vi "NI-USB6343.vi"() -> ()   [LabVIEW 2020]
doc: "test"
uses:
  LabVIEW 2020 Toolkits/toolkits_lv2020_32bit/Synchronization.llb/SynchRefs_SetGet.ctl
  LabVIEW 2020 Toolkits/VI Server Toolkit/VI Server Libraries/VI Server_SetControl.llb/VI Server_BOOL_Set.vi
  LabVIEW 2020 Toolkits/VI Server Toolkit/VI Server Libraries/VI Server_Set Controls.llb/Set STR Control.vi
  LabVIEW 2020 Toolkits/VI Server Toolkit/VI Server Libraries/VI Server_GetControl.llb/VI Server_STR_Get.vi
  LabVIEW 2020 Toolkits/VI Server Toolkit/VI Server Libraries/VI Server_GetControl.llb/VI Server_DAQmx_Device_Get.vi
  LabVIEW 2020 Toolkits/VI Server Toolkit/VI Server Toolkit LV2013.lvlib
panel:
  in  "LastAction.AddToSecuence":bool
  out "System.Message":string caption="System Message"
  in  "Help":bool
  in  "FP.Hide":bool caption="FrontPanel.Hide"
  in  "EXIT":bool
  in  "Tab.Main":T1(tab)
  in  "AI.SaveGraphToFile":bool
  in  "AI.Graph.Plots":u16(ring) items=["NI-USB6343/ai0", "NI-USB6343/ai1", "NI-USB6343/ai2"]
  out "AI.WaveformGraph":waveform(dbl)[](graph) caption="Waveform Graph"
  in  "AI.MultiChannelAcquisition":bool
  in  "AI.PhysicalChannel.Include":bool
  out "AI.ActualSampleRate":dbl=1000.0 caption="Actual Sample Rate" format="%0.2f"
  out "AI.Averaged.Mesurement":dbl caption="Averaged Mesurement" format="%0.4f V"
  in  "AI.Measure":bool caption="AI:Measure"
  in  "AI.Number.Of.Samples":i32=100 caption="Number Of Samples"
  in  "AI.SampleRate":dbl=1000.0 caption="Sample Rate" format="%0.0f Hz"
  in  "AI.MinInputLimit":dbl caption="Min Input Limit" min=-10.0 max=10.0 format="%0.3f V"
  in  "AI.MaxInputLimit":dbl caption="Max Input Limit" min=-10.0 max=10.0 format="%0.3f V"
  in  "AI.TerminalConfiguration":u16(ring)=65535 caption="Terminal Configuration" items=["default"=65535, "RSE"=10083, "NRSE"=10078, "Differential"=10106, "Pseudodifferential"=12529]
  in  "AI.Sample.Mode":u16(ring)=12522 caption="Sample Mode" items=["Finite Samples"=10178, "Continuous Samples"=10123]
  in  "AI.Physical.Channel":tag="Dev1/ai0" caption="Physical Channel"
  out "AO.Update.Time":u32 caption="AO Update Time" format="%.0f msec"
  in  "AO.GenerationMode":u16(ring) caption="Generation Mode" items=["Voltage DC", "Voltage Sine Wave Generation", "Voltage Triangle Wave Generation", "Voltage Square Wave Generation", "Voltage Sawtooth Wave Generation"]
  in  "AO.Physical.Channel":tag="Dev1/ai0" caption="Physical Channel"
  in  "AO.Update":bool
  in  "AO.Output":bool caption="AO:Output"
  in  "AO.SampleMode":u16(ring) caption="Sample Mode" items=["Finite Samples"=10178, "Continious Samples"=10123]
  in  "AO.NumberOfSamples":i32=1000 caption="Number Of Samples" min=2
  in  "AO.SampleRate":dbl=1000.0 caption="Sample Rate" format="%0.1f Hz"
  in  "AO.Sample.Clock.Source":tag="OnboardClock" caption="Sample Clock Source"
  out "AO.ActualSampleRate":dbl=1000.0 caption="Actual Sample Rate" format="%0.2f"
  in  "AO.MaxVoltage":dbl=5.0 caption="Max Voltage" format="%0.3f V"
  in  "AO.MinVoltage":dbl=-5.0 caption="Min Voltage" format="%0.3f V"
  out "AO.WaveformGraph":waveform(dbl)(graph) caption="Waveform Graph"
  in  "AO.OutputVoltage":dbl(slide) caption="Amplitude" min=-10.0 max=10.0 scale=-10.0..10.0 scale format="%0.3f V"
  in  "AO.SinewaveFrequency":dbl=10.0 caption="Sinewave Frequency" format="%0.2p Hz"
  in  "DO.Port.Mask.Apply":bool caption="DO:Port.Mask.Apply"
  in  "DO.Port.Lines.31:24.Mask":u8 caption="Port&Lines 31:24" format="%08b"
  in  "DO.Port.Lines.23:16.Mask":u8 caption="Port&Lines 23:16" format="%08b"
  in  "DO.Port.Lines.15:8.Mask":u8 caption="Port&Lines 15:8" format="%08b"
  in  "DO.Port.Lines.7:0.Mask":u8 caption="Port&Lines 7:0" format="%08b"
  out "DO.Port.State.Verify":bool caption="Verified"
  out "DO.Line.State.Verify":bool caption="Verified"
  in  "DO.Line.State":bool caption="State"
  in  "DO.Line":tag="Dev1/port0/line0:7" caption="Line"
  in  "DO.Line.Update":bool caption="Update:"
  in  "DO.Port.Update":bool caption="DO:Port.Update"
  in  "DO.Port.Lines.31:24":u8 caption="Port&Lines 31:24" format="%08b"
  in  "DO.Port.Lines.23:16":u8 caption="Port&Lines 23:16" format="%08b"
  in  "DO.Port.Lines.15:8":u8 caption="Port&Lines 15:8" format="%08b"
  in  "DO.Port.Lines.7:0":u8 caption="Port&Lines 7:0" format="%08b"
  in  "DO.Port":tag="Dev1/port0/line0:7" caption="Port"
  out "DI.Line.State":bool caption="State"
  in  "DI.Port.Update":bool caption="DI:Port.Update"
  out "DI.Port.Lines.24:31":u8 caption="Port&Lines 31:24" format="%08b"
  out "DI.Port.Lines.16:23":u8 caption="Port&Lines 23:16" format="%08b"
  out "DI.Port.Lines.8:15":u8 caption="Port&Lines 15:8" format="%.0b"
  out "DI.Port.Lines.0:7":u8 caption="Port&Lines 7:0" format="%08b"
  in  "DI.Port":tag="Dev1/port0/line0:7" caption="Port"
  in  "DI.Line":tag="Dev1/port0/line0:7" caption="Line"
  in  "DI.Line.Update":bool caption="Update:"
  out "ctr3.Out.Duty Cycle.Actual":dbl caption="Ctr3: Duty Cycle Actual" format="%.2f"
  out "ctr3.Out.Frequency.Actual":dbl caption="Ctr3: Frequency Actual" format="%0.3f Hz"
  out "ctr2.Out.Duty Cycle.Actual":dbl caption="Ctr2: Duty Cycle Actual" format="%.2f"
  out "ctr2.Out.Frequency.Actual":dbl caption="Ctr2: Frequency Actual" format="%0.3f Hz"
  out "ctr1.Out.Duty Cycle.Actual":dbl caption="Ctr1: Duty Cycle Actual" format="%.2f"
  out "ctr1.Out.Frequency.Actual":dbl caption="Ctr1: Frequency Actual" format="%0.3f Hz"
  out "ctr0.Out.Duty Cycle.Actual":dbl caption="Ctr0: Duty Cycle Actual" format="%.2f"
  out "ctr0.Out.Frequency.Actual":dbl caption="Ctr0: Frequency Actual" format="%0.3f Hz"
  in  "Cntr.Out.NumberOfPulses":i32=1000 caption="Number Of Pulses" min=1
  in  "Cntr.Out.Start":bool
  in  "Cntr.Out.Sample.Mode":u16(ring)=10123 caption="Sample Mode" items=["Finite Samples"=10178, "Continuous Samples"=10123, "Hardware Timed Single Point"=12522]
  in  "Cntr.Out.Duty.Cycle":dbl=0.5 caption="Duty Cycle" format="%.2f %"
  in  "Cntr.Out.Frequency":dbl=1.0 caption="Frequency" format="%0.3f Hz"
  in  "Cntr.Out.Output.Terminal":tag="/Dev1/PFI12" caption="Output Terminal"
  in  "Cntr.Out.Channel":tag="Dev1/ctr0" caption="Channel"
  out "ctr3.In.Count":u32 caption="Count.3:"
  out "ctr2.In.Count":u32 caption="Count.2:"
  out "ctr1.In.Count":u32 caption="Count.1:"
  out "ctr0.In.Count":u32 caption="Count.0:"
  in  "Cntr.In.Start":bool
  in  "Cntr.In.IntegrationTime":u32=10 format="%.0f msec"
  in  "Cntr.In.Sample.Clock.Source":tag="PFI0" caption="Sample Clock Source"
  in  "Cntr.In.ActiveEdge":u16(ring)=10280 caption="Active Edge" items=["Rising"=10280, "Falling"=10171]
  in  "Cntr.In.Input.Terminal":tag="PFI8" caption="Input.Terminal"
  in  "Cntr.In.Channel":tag="Dev1/port0/line0:7" caption="Channel Name"
  in  "Settings.LOAD":bool
  in  "Settings.SAVE":bool
  in  "Settings.Number":i32=1 caption="Number" min=1 step=1
  in  "Settings.Type":u16(ring) caption="Type" items=["AI", "AO", "Dig I/O", "Counter In", "Counter Out"]
  in  "TestCase.Execute.All":bool
  in  "TestCase.Execute.Selected":bool
  out "TestCase.SAVE.Success":bool
  in  "TestCase.SAVE":bool
  in  "SequenceFile.Open":bool
  in  "SequenceFile":path caption="Secuence File"
  in  "TestCase.Execute.Step.Pause":bool
  in  "TestCase.Execute.Steps":u16(ring) caption="Test Case: Pause Before Step" items=["1", "2", "3", "4", "5", "6", "7", "8", "9", "10"]
  in  "TestCase.Execute.ABORT":bool
  in  "TestCase.Execute.Next":bool
  in  "TestCase.Execute.Pause":bool
  out "TestCase.ExecutionTime":dbl caption="Execution Time:" format="%0.3f sec"
  in  "TestCase.Execution.StepTime":u32 caption="Seq. Execution: Step Time" format="%d msec"
  in  "TestCaseConfiguration":i32[](listbox) caption="Test Case Configuration"
  in  "TestCase.StepDescription":string caption="Step Description:"
  in  "DisableFP_OpenOnIDN_Call":bool caption="Disable FP Open\nON *IDN? Call"
  in  "DisableFP_Hide":bool caption="Disable FP Hide"
  in  "UDP.Test.String1.SendLocal":bool caption="UDP.Test.String1.Send"
  in  "ProductType":string="USB-6343 (BNC)" caption="Product Type"
  in  "VI.WindowsTitle":string caption="Windows Title"
  in  "DAQmx.Device":tag caption="DAQmx: Device"
  in  "Cont.Measurements.CycleTime":u32 caption="Continius Measurements:\nCycleTime"
  in  "UDP.Test.String2.Send":bool
  in  "UDP.Test.String2":string caption="UDP: Test String 2"
  in  "UDP.Port.BC":u16=58433 caption="UDP: Port.BC"
  in  "UDP.Port.RT":u16=58432 caption="UDP: Port.RT"
  in  "UDP.LocalPort":u16=58434 caption="UDP: Local Port"
  in  "UDP.IP.Address":string="234.5.6.7" caption="UDP: IP Address"
  in  "UDP.Test.String1.Send.ToInstr":bool caption="UDP.Test.String1.Send"
  in  "UDP.Test.String1":string caption="UDP: Test String 1"
  in  "UDP.Responce.String.Monitor":bool
  out "UDP.ExecEng.Message.String":string caption="UDP: Execution Engine Message String"
  out "error out":errorcluster={"status"=TRUE, "code"=1055, "source"="Property Node in VI Server Toolkit LV2013.lvlib:VI server_Set Control Value from String Format.vi:5200001->DMM6500_UDP_ExecEng_Instruction_APPLY.vi->DMM6500_UDP_MAIN.vi->Keithley2100.vi"}
  in  "error in":errorcluster
  # "Important Note: Analog Input configuration shall\nstart from Physical Channel selection!"
  # "Important Note: Analog Output configuration shall\nstart from Physical Channel selection!"
  # "Analog Output Configuration (Generic)"
  # "Digital Output Port\nMASK"
  # "Instructions:\n1: Active Bit; 0: Masked Bit"
  # "Digital Output"
  # "Digital Input"
  # "Counter Input"
  # "Counter Input"
  # "Counter Output"
  # "Settings"
  # "M"
  # "Multicast IP addresses must be in the 224.0.0.0 to 239.255.255.255 range."
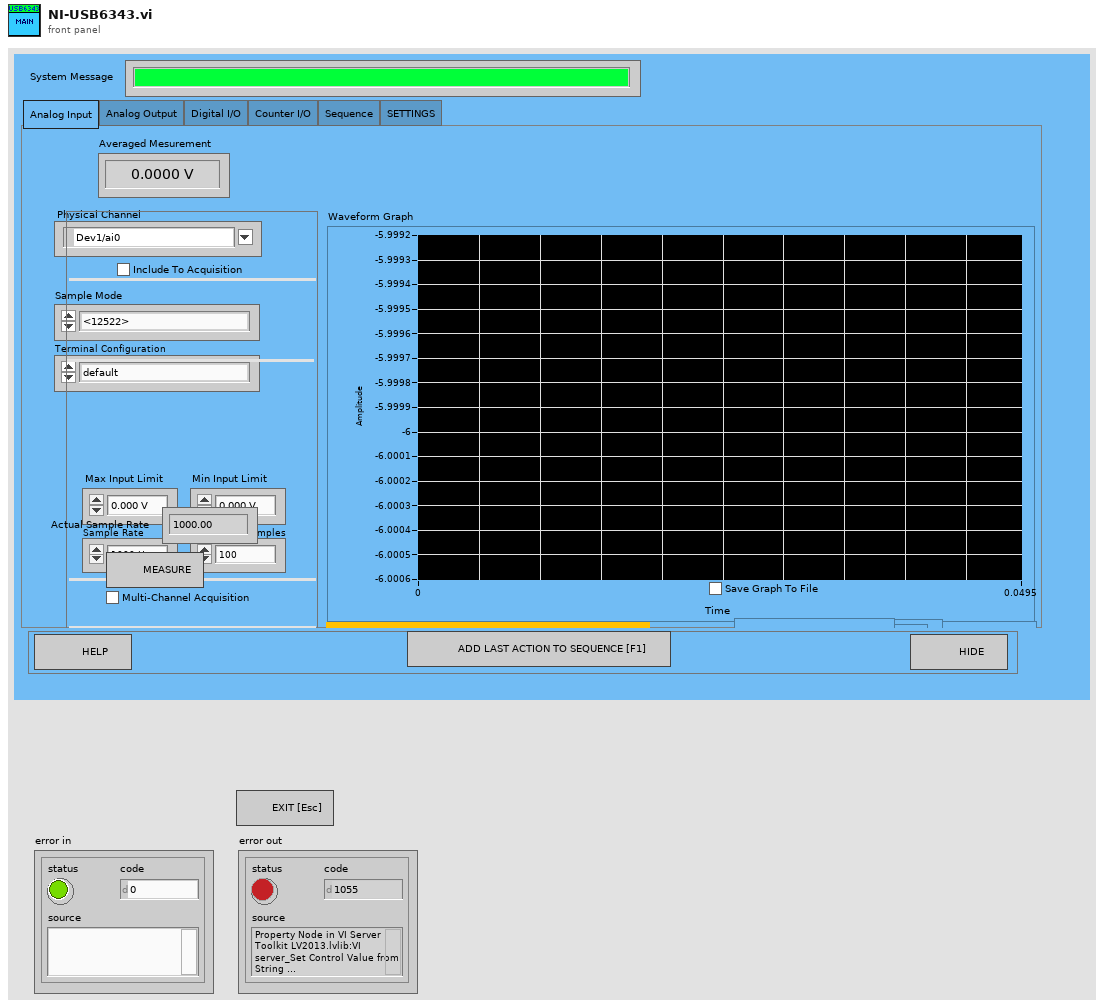
[diagram p1: front panel]
types:
  T1 = enum32{"Analog Input", "Analog Output", "Digital I/O", "Counter I/O", "Sequence", "SETTINGS"}
  T2 = typedef "VI Server_RefsCluster.ctl" = cluster{"Labels":string[], "Refs":refnum<vi>[], "VI Ref":refnum<vi>}
  T3 = typedef "SynchRefs_SetGet.ctl" = enum16{"Set", "Get"}
  T4 = enum8{"Enabled", "Disabled", "Disabled and Grayed Out"}
  T5 = cluster{"Color":u32, "PointStyle":u8, "LineStyle":u8, "Interp":u8, "LineWidth":u8, "BarPlotStyle":u8, "FillTo":i16, "XScaleIdx":u32, "YScaleIdx":u32, "Anti-Aliased":bool, "LabelFormat":u8, "TransitionType":u8, "TransitionLocation":u8, "DigitalLineStyle":u8}
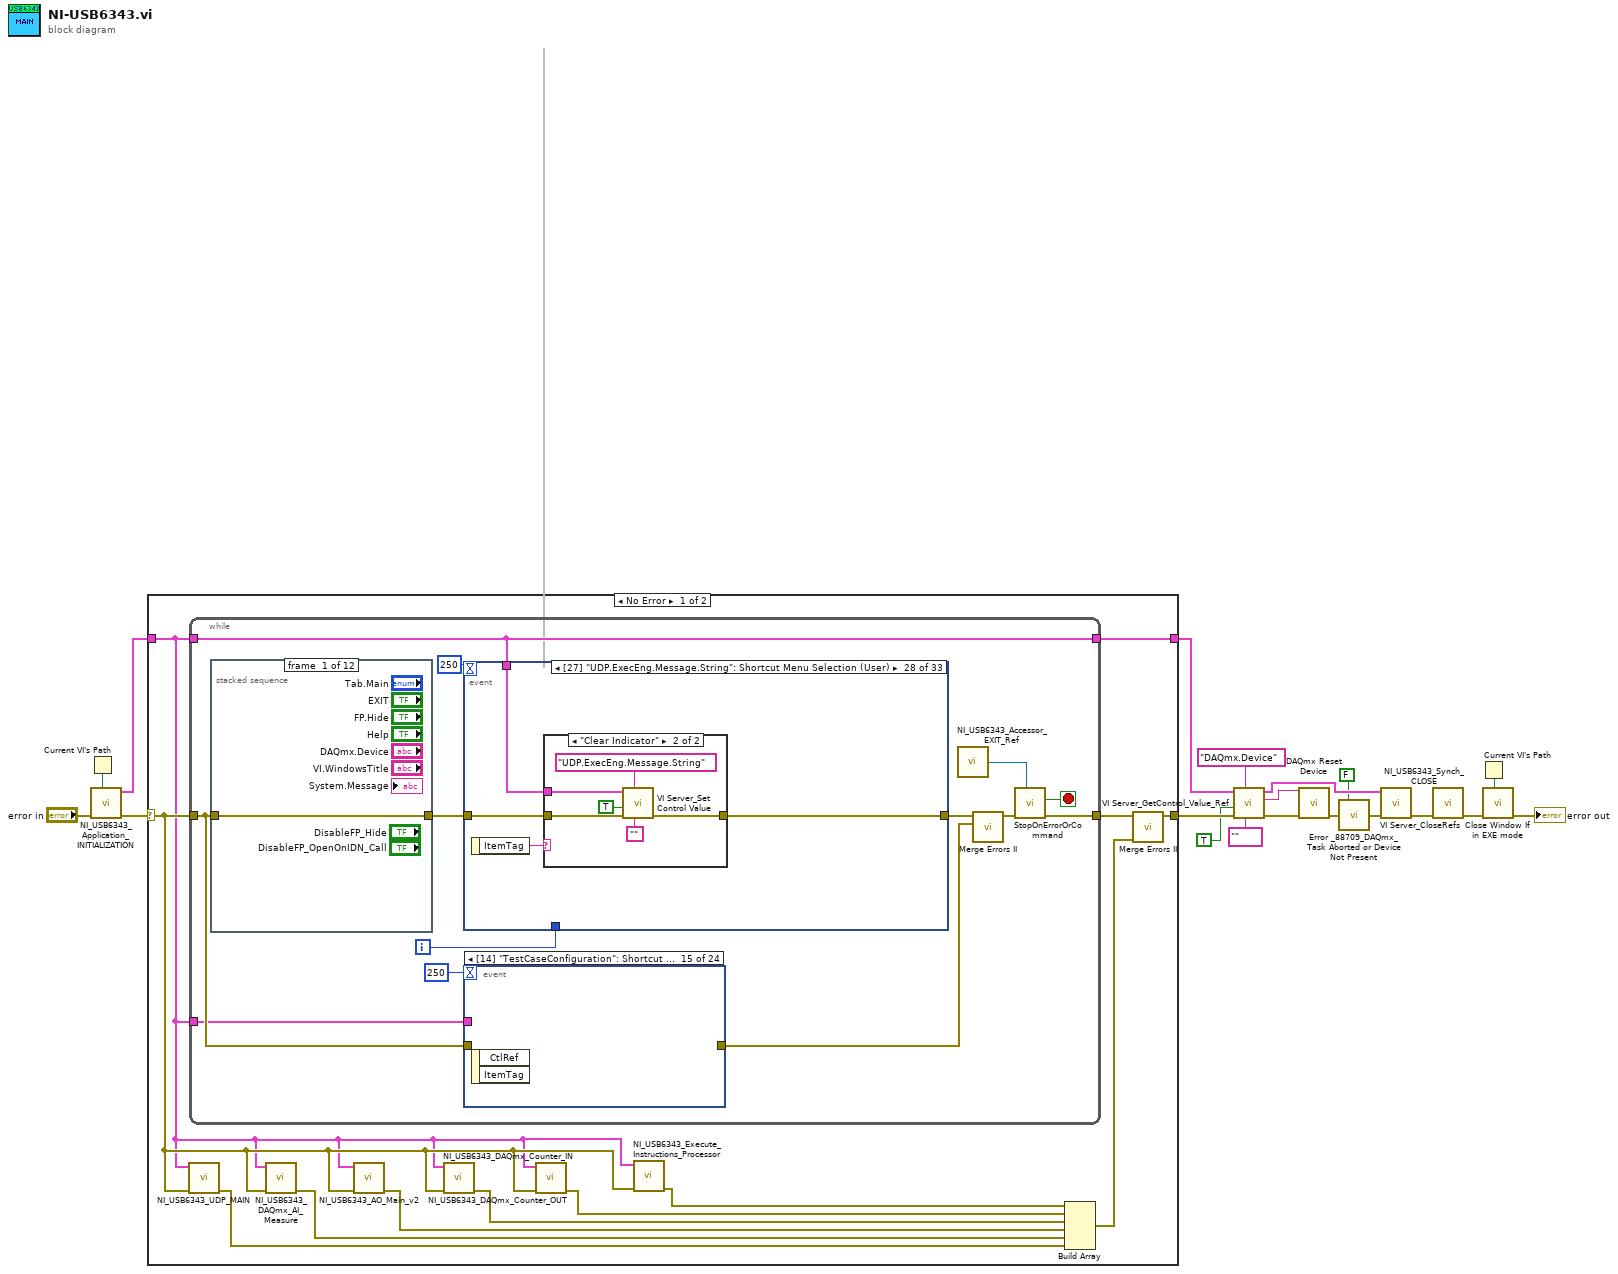
[diagram p0: block diagram]
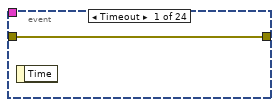
[diagram p2: hidden frame]
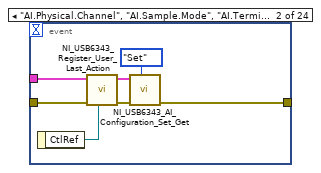
[diagram p3: hidden frame]
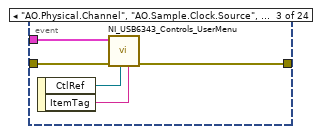
[diagram p4: hidden frame]
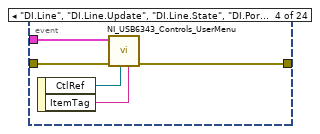
[diagram p5: hidden frame]
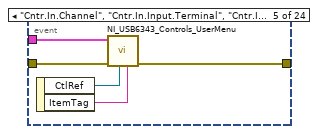
[diagram p6: hidden frame]
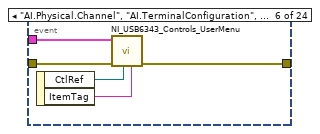
[diagram p7: hidden frame]
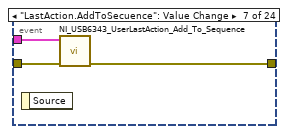
[diagram p8: hidden frame]
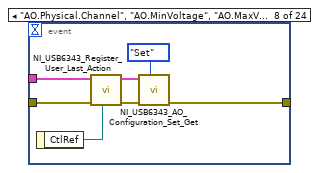
[diagram p9: hidden frame]
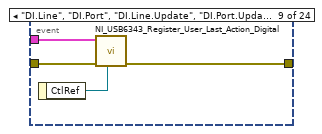
[diagram p10: hidden frame]
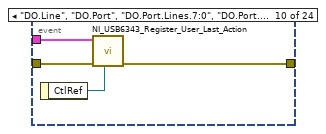
[diagram p11: hidden frame]
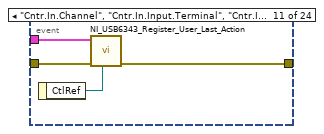
[diagram p12: hidden frame]
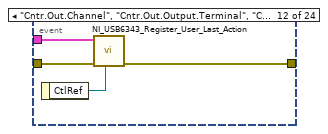
[diagram p13: hidden frame]
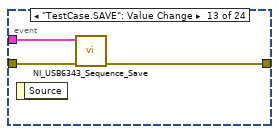
[diagram p14: hidden frame]
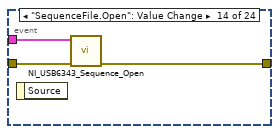
[diagram p15: hidden frame]
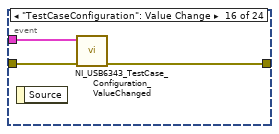
[diagram p16: hidden frame]
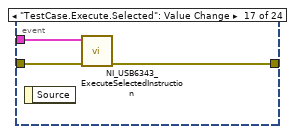
[diagram p17: hidden frame]
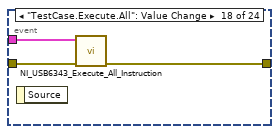
[diagram p18: hidden frame]
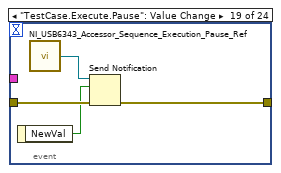
[diagram p19: hidden frame]
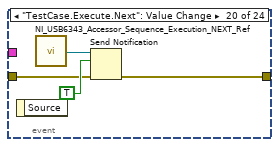
[diagram p20: hidden frame]
diagram:
  n1 = Current VI's Path() -> (path=w3:path)
  n2 = call "NI_USB6343_Application_INITIALIZATION.vi"("Top VI Path"=w3, "error in (no error)"="error in") -> ("error out"=w19:errorcluster, "VI Server Cluster.OUT"=w2:T2)  [unwired: 8 in]
  n3 = case shown="No Error" w19 {
    selector: w19 -> [w22 w366]
    tunnel: [w28 w366] -> w13
    tunnel: w2 -> [w20 w365]
    tunnel: [w31 w365] -> w11
    frame No Error {
      n4 = call "NI_USB6343_UDP_MAIN.vi"("error in (no error)"=w22, "VI Server.RefsCluster"=w20) -> ("error out"=w30:errorcluster)  [unwired: 9 in]
      n5 = while {
        tunnel: w22 -> [w36]
        tunnel: [w40] -> w29
        tunnel: w20 -> [w41]
        tunnel: [w41] -> w31
        tunnel: w20 -> [w32]
        i -> [w42]
        stop <- w39 stop-if-true
        n6 = stacked-sequence {
          tunnel: w36 -> [w364 _ _ _ _ _ _ _ _ _ _ _]
          tunnel: [w364 _ _ _ _ _ _ _ _ _ _ _] -> w44
          frame #0 {
          }
          frame #1 {
          }
          frame #2 {
          }
          frame #3 {
          }
          frame #4 {
          }
          frame #5 {
          }
          frame #6 {
          }
          frame #7 {
          }
          frame #8 {
          }
          frame #9 {
          }
          frame #10 {
          }
          frame #11 {
          }
        }
        n7 = event shown="[27] \"UDP.ExecEng.Message.String\": Shortcut Menu Selection (User)" {
          selector: _ -> [_ _ _ _ _ _ _ _ _ _ _ _ _ _ _ _ _ _ _ _ _ _ _ _ _ _ _ _ _ _ _ _ _]
          dyn-events: _ -> [_ _ _ _ _ _ _ _ _ _ _ _ _ _ _ _ _ _ _ _ _ _ _ _ _ _ _ _ _ _ _ _ _]
          timeout: 250 -> [_ _ _ _ _ _ _ _ _ _ _ _ _ _ _ _ _ _ _ _ _ _ _ _ _ _ _ _ _ _ _ _ _]
          tunnel: w44 -> [w146 w160 w163 w169 w178 w193 w200 w213 w225 w232 w235 w240 w251 w257 w263 w266 w270 w273 w277 w280 w284 w293 w300 w303 w304 w314 w316 w320 w331 w340 w349 w358 w362]
          tunnel: w42 -> [_ _ _ _ _ _ _ _ _ _ _ _ _ _ _ _ _ _ _ _ _ _ _ _ _ _ _ _ _ _ _ _ w361]
          tunnel: [w148 w158 w164 w171 w176 w191 w198 w210 w226 w230 w236 w238 w245 w256 w260 w265 w268 w271 w275 w278 w283 w290 w298 w301 w306 w309 w316 w318 w329 w338 w347 w356 w359] -> w35
          tunnel: w41 -> [w145 _ w165 w167 _ w189 w199 w212 w223 w231 w234 w239 w250 w255 w262 w264 w269 w272 _ w279 w282 _ w299 w302 _ w313 _ w317 _ w337 w346 w355 w360]
          event "AI.Physical.Channel": Value Change {
            n8 = event-data() -> ("OldVal"=w143:tag, "NewVal"=w141:tag)  [unwired: 1 in]
            n9 = call "NI_USB6343_AI_CheckPhysicalChannel.vi"("NewVal"=w141, "OldVal"=w143, "error in (no error)"=w146, "VI Server Cluster"=w145) -> ("error out"=w147:errorcluster, "AI.Settings.Update"=w142:bool, "VI Server Cluster DUP"=w144:T2)  [unwired: 5 in]
            n10 = case shown="True" w142 {
              tunnel: [w149 w152] -> w148
              tunnel: w147 -> [w149 w155]
              tunnel: w144 -> [_ w154]
              tunnel: w141 -> [_ w151]
              frame False {
              }
              frame True {
                n11 = Type Cast(x=w151) -> (*(type *) &x=w150:string)  [unwired: 1 in]
                n12 = call "NI_USB6343_AI_Configuration_Set_Get.vi"("SynchRefs.Set/Get"=SynchRefs_SetGet."Get", "error in (no error)"=w155, "VI Server Cluster"=w154) -> ("error out"=w153:errorcluster)  [unwired: 6 in, 2 out]
                n13 = property on="AI.WaveformGraph" class="WFGraph (strict)"(error in=w153, "Plot.Plot Name"=w150) -> (error out=w152:errorcluster)  [unwired: 1 in, 1 out]
              }
            }
          }
          event "AI.SaveGraphToFile": Value Change {
            n14 = event-data() -> ("NewVal"=w157:bool)  [unwired: 1 in]
            n15 = call "NI_USB6343_Accessor_AI_SaveGraphToFile_Ref.vi"() -> ("AI.SaveGraphToFile"=w159:refnum<notifier>)  [unwired: 6 in]
            n16 = Send Notification(notification=w157, notifier=w159, error in (no error)=w160) -> (error out=w158:errorcluster)  [unwired: 1 out]
          }
          event "AI.WaveformGraph": Plot Attribute Change {
            n17 = event-data() -> ("OldAttrib"=w162:T5, "NewAttrib"=w161:T5)  [unwired: 1 in]
            n18 = call "NI_USB6343_AI_Graph_PlotAttribute_ValueChanged.vi"("NewAttrib"=w161, "OldAttrib"=w162, "error in (no error)"=w163, "VI Server Cluster"=w165) -> ("error out"=w164:errorcluster)  [unwired: 7 in]
          }
          event "AO.GenerationMode": Value Change {
            n19 = event-data() -> ("NewVal"=w175:u16)  [unwired: 1 in]
            n20 = call "NI_USB6343_AO_Configuration_Set_Get.vi"("SynchRefs.Set/Get"=SynchRefs_SetGet."Set", "error in (no error)"=w169, "VI Server Cluster"=w167) -> ("error out"=w170:errorcluster, "VI Server Cluster.DUP"=w168:T2)  [unwired: 6 in, 1 out]
            n21 = call "NI_USB6343_AO_GenerationMode.vi"("AO.GenerationMode"=w175, "error in (no error)"=w170, "VI Server Cluster"=w168) -> ("error out"=w172:errorcluster)  [unwired: 7 in, 1 out]
            n22 = call "NI_USB6343_Accessor_ao_Waveform_Array_Update_Ref.vi"() -> ("ao.Waveform.Array.Update"=w174:refnum<notifier>)  [unwired: 6 in]
            n23 = Send Notification(notification=TRUE, notifier=w174, error in (no error)=w172) -> (error out=w171:errorcluster)  [unwired: 1 out]
          }
          event "AO.Output": Value Change {
            n24 = event-data() -> ("NewVal"=w177:bool)  [unwired: 1 in]
            n25 = disable-structure shown="Enabled" {
              disable-tunnel: w178 -> [w185 w186]
              disable-tunnel: w177 -> [w183 _]
              disable-tunnel: [w180 w186] -> w176
              frame Enabled {
                n26 = call "NI_USB6343_Accessor_ao0_State_Ref.vi"() -> ("ao0.State"=w184:refnum<notifier>)  [unwired: 6 in]
                n27 = Send Notification(notification=w183, notifier=w184, error in (no error)=w185) -> (error out=w181:errorcluster)  [unwired: 1 out]
                n28 = call "NI_USB6343_Accessor_ao_Waveform_Array_Update_Ref.vi"() -> ("ao.Waveform.Array.Update"=w182:refnum<notifier>)  [unwired: 6 in]
                n29 = Send Notification(notification=TRUE, notifier=w182, error in (no error)=w181) -> (error out=w180:errorcluster)  [unwired: 1 out]
              }
              frame Disabled {
              }
            }
          }
          event "AO.Physical.Channel": Value Change {
            n30 = event-data() -> ("NewVal"=w187:tag)  [unwired: 1 in]
            n31 = call "NI_USB6343_AO_Configuration_Set_Get.vi"("SynchRefs.Set/Get"=SynchRefs_SetGet."Get", "error in (no error)"=w193, "VI Server Cluster"=w189) -> ("error out"=w190:errorcluster, "VI Server Cluster.DUP"=w188:T2)  [unwired: 6 in, 1 out]
            n32 = call "NI_USB6343_AO_PhysicalChannel_UpdateGraph.vi"("AO.Physical.Channel"=w187, "error in (no error)"=w190, "VI Server Cluster"=w188) -> ("error out"=w191:errorcluster)  [unwired: 8 in]
          }
          event "AO.Sample.Clock.Source", "AO.SampleMode", "AO.SampleRate", "AO.NumberOfSamples", "AO.MaxVoltage", "AO.MinVoltage": Value Change {
            n33 = event-data() -> ()  [unwired: 1 in, 1 out]
            n34 = call "NI_USB6343_AO_ConfigurationAtributes.vi"("error in (no error)"=w200, "VI Server Cluster"=w199) -> ("error out"=w197:errorcluster)  [unwired: 8 in, 1 out]
            n35 = call "NI_USB6343_Accessor_ao0_State_Ref.vi"() -> ("ao0.State"=w195:refnum<notifier>)  [unwired: 6 in]
            n36 = Get Notifier Status(notifier=w195, error in (no error)=w197) -> (current notification=w194:bool, error out=w196:errorcluster)  [unwired: 3 out]
            n37 = case shown="True" w194 {
              tunnel: [w201 w206] -> w198
              tunnel: w196 -> [w201 w203]
              tunnel: w195 -> [_ w202]
              frame False {
              }
              frame True {
                w205 = TRUE ("notification")
                n38 = Send Notification(notification=FALSE, notifier=w202, error in (no error)=w203) -> (error out=w208:errorcluster)  [unwired: 1 out]
                n39 = call "NI_USB6343_Accessor_ao_Waveform_Array_Update_Ref.vi"() -> ("ao.Waveform.Array.Update"=w209:refnum<notifier>)  [unwired: 6 in]
                n40 = Send Notification(notification=w205, notifier=w209, error in (no error)=w208) -> (error out=w207:errorcluster)  [unwired: 1 out]
                n41 = Send Notification(notification=w205, notifier=w202, error in (no error)=w207) -> (error out=w206:errorcluster)  [unwired: 1 out]
              }
            }
          }
          event "AO.SinewaveFrequency", "AO.OutputVoltage": Value Change {
            n42 = event-data() -> ()  [unwired: 1 in, 4 out]
            n43 = call "VI Server_CycleEventBySignalingValue.vi"("Label"="AO.GenerationMode", "error in"=w213, "VI Server.RefsCluster"=w212) -> ("error out"=w210:errorcluster)  [unwired: 7 in, 1 out]
          }
          event "AO.Update": Value Change {
            w216 = TRUE ("Single Instance (T)")
            n44 = event-data() -> ()  [unwired: 1 in, 1 out]
            n45 = call "VI Server_Get Text Ring Selection.vi"("Label"="AO.GenerationMode", "error in"=w225, "Single Instance (T)"=w216, "VI Server Cluster"=w223) -> ("error out"=w221:errorcluster, "VI Server Custer.DUP"=w222:T2, "Value"=w220:u16)  [unwired: 2 in, 3 out]
            n46 = call "NI_USB6343_AO_GenerationMode.vi"("AO.GenerationMode"=w220, "error in (no error)"=w221, "VI Server Cluster"=w222) -> ("error out"=w219:errorcluster, "VI Server Cluster.DUP"=w217:T2)  [unwired: 7 in]
            n47 = call-poly "VI Server_SetControl.vi"("Data"=FALSE, "Control.Label"="AO.Update" ("Label"), "error in"=w219, "SingleInstance"=w216, "VI Server.RefsCluster"=w217) -> ("error out"=w218:errorcluster)  [unwired: 4 in, 2 out]
            n48 = call "NI_USB6343_Accessor_ao_Waveform_Array_Update_Ref.vi"() -> ("ao.Waveform.Array.Update"=w228:refnum<notifier>)  [unwired: 6 in]
            n49 = Send Notification(notification=TRUE, notifier=w228, error in (no error)=w218) -> (error out=w226:errorcluster)  [unwired: 1 out]
          }
          event "Cntr.In.Channel": Value Change {
            n50 = event-data() -> ("NewVal"=w229:tag)  [unwired: 1 in]
            n51 = call "NI-USB6343_Counter_IN_GetStateFromFile.vi"("Counter.IN.Channel"=w229, "error in (no error)"=w232, "VI Server Cluster"=w231) -> ("error out"=w230:errorcluster)  [unwired: 7 in, 1 out]
          }
          event "Cntr.In.Start": Value Change {
            n52 = event-data() -> ("NewVal"=w233:bool)  [unwired: 1 in]
            n53 = call "NI-USB6343_Counter_IN_SaveStateToFile.vi"("Cntr.In.Start"=w233, "error in (no error)"=w235, "VI Server Cluster"=w234) -> ("error out"=w236:errorcluster)  [unwired: 7 in, 1 out]
          }
          event "Cntr.Out.Channel": Value Change {
            n54 = event-data() -> ("NewVal"=w241:tag, "OldVal"=w237:tag)  [unwired: 1 in]
            n55 = call "NI-USB6343_Counter_OUT_GetStateFromFile.vi"("Counter.OUT.Channel.Old"=w237, "Counter.OUT.Channel.New"=w241, "error in (no error)"=w240, "VI Server Cluster"=w239) -> ("error out"=w238:errorcluster)  [unwired: 6 in, 1 out]
          }
          event "Cntr.Out.Sample.Mode": Value Change {
            n56 = event-data() -> ()  [unwired: 1 in, 1 out]
            n57 = call "VI Server_Get Text Ring Selection.vi"("Label"="Cntr.Out.Sample.Mode", "error in"=w251, "Single Instance (T)"=TRUE, "VI Server Cluster"=w250) -> ("error out"=w246:errorcluster, "Selection"=w247:string, "VI Server Custer.DUP"=w244:T2)  [unwired: 2 in, 3 out]
            n58 = case shown="\"Finite Samples\"" w247 {
              tunnel: [T4."Disabled and Grayed Out" ("Disabled") T4."Enabled" ("Disabled")] -> w243
              frame "Continuous Samples", Default {
              }
              frame "Finite Samples" {
              }
            }
            n59 = call "VI Server_Enable_Disable.vi"("Disabled"=w243, "Label"="Cntr.Out.NumberOfPulses", "error in"=w246, "VI Server Cluster"=w244) -> ("error out"=w245:errorcluster)  [unwired: 5 in, 2 out]
          }
          event "Cntr.Out.Start": Value Change {
            n60 = event-data() -> ("NewVal"=w254:bool)  [unwired: 1 in]
            n61 = call "NI-USB6343_Counter_OUT_SaveStateToFile.vi"("Cntr.In.Start"=w254, "error in (no error)"=w257, "VI Server Cluster"=w255) -> ("error out"=w256:errorcluster)  [unwired: 7 in, 1 out]
          }
          event "DAQmx.Device": Value Change {
            n62 = event-data() -> ("NewVal"=w258:tag)  [unwired: 1 in]
            n63 = call "NI_USB6343_DAQmx_LimitPhysicalChannelsToDevice.vi"("error in (no error)"=w263, "VI Server Cluster"=w262) -> ("error out"=w261:errorcluster, "VI Server Cluster.DUP"=w259:T2)  [unwired: 7 in, 1 out]
            n64 = call "NI_USB6343_DAQmx_DeviceName_Changed_UpdateSet_Get_Sections.vi"("DAQmx.Device"=w258, "error in (no error)"=w261, "VI Server Cluster"=w259) -> ("error out"=w260:errorcluster)  [unwired: 8 in]
          }
          event "DI.Line.Update": Value Change {
            n65 = event-data() -> ()  [unwired: 1 in, 1 out]
            n66 = call "NI_USB6343_Digital_Input_Line_Update.vi"("error in (no error)"=w266, "VI Server Cluster"=w264) -> ("error out"=w265:errorcluster)  [unwired: 9 in]
          }
          event "DI.Port": Value Change {
            n67 = event-data() -> ("NewVal"=w267:tag)  [unwired: 1 in]
            n68 = call "NI_USB6343_DI_Port_ValueChanged.vi"("DI.Port"=w267, "error in (no error)"=w270, "VI Server Cluster"=w269) -> ("error out"=w268:errorcluster)  [unwired: 8 in]
          }
          event "DI.Port.Update": Value Change {
            n69 = event-data() -> ()  [unwired: 1 in, 1 out]
            n70 = call "NI_USB6343_DI_Port_Update.vi"("error in (no error)"=w273, "VI Server Cluster"=w272) -> ("error out"=w271:errorcluster)  [unwired: 9 in]
          }
          event "DisableFP_Hide": Value Change {
            n71 = event-data() -> ("NewVal"=w274:bool)  [unwired: 1 in]
            n72 = call "NI_USB6343_Accessor_DisableFP_Hide_Ref.vi"() -> ("DisableFP_Hide"=w276:refnum<notifier>)  [unwired: 6 in]
            n73 = Send Notification(notification=w274, notifier=w276, error in (no error)=w277) -> (error out=w275:errorcluster)  [unwired: 1 out]
          }
          event "DO.Line.Update": Value Change {
            n74 = event-data() -> ()  [unwired: 1 in, 1 out]
            n75 = call "NI_USB6343_Digital_Output_Line_Update.vi"("error in (no error)"=w280, "VI Server Cluster"=w279) -> ("error out"=w278:errorcluster)  [unwired: 9 in]
          }
          event "DO.Port": Value Change {
            n76 = event-data() -> ("NewVal"=w281:tag)  [unwired: 1 in]
            n77 = call "NI_USB6343_DO_Port_ValueChanged.vi"("DO.Port"=w281, "error in (no error)"=w284, "VI Server Cluster"=w282) -> ("error out"=w283:errorcluster)  [unwired: 8 in]
          }
          event "DO.Port.Lines.7:0", "DO.Port.Lines.15:8", "DO.Port.Lines.23:16", "DO.Port.Lines.31:24", "DO.Port.Lines.7:0.Mask", "DO.Port.Lines.15:8.Mask", "DO.Port.Lines.23:16.Mask", "DO.Port.Lines.31:24.Mask", "DI.Port.Lines.0:7", "DI.Port.Lines.8:15", "DI.Port.Lines.16:23", "DI.Port.Lines.24:31": Mouse Down {
            n78 = event-data() -> ("CtlRef"=w292:refnum<vi>)  [unwired: 1 in]
            n79 = property class="DigNum (strict)"(reference=w292, error in=w293) -> (reference out=w289:refnum<vi>, error out=w291:errorcluster, "FormatString"=w286:string)
            n80 = Match Pattern(string=w286, regular expression="[0-9]+") -> (after substring=w285:string)  [unwired: 1 in, 3 out]
            n81 = case shown="\"b\", Default" w285 {
              tunnel: ["%.0f" "%02x" "%02o" "%08b"] -> w288
              frame "f" {
              }
              frame "x" {
              }
              frame "o" {
              }
              frame "b", Default {
              }
            }
            n82 = property class="DigNum (strict)"(reference=w289, error in=w291, "FormatString"=w288) -> (error out=w290:errorcluster)  [unwired: 1 out]
          }
          event "DO.Port.Mask.Apply": Value Change {
            n83 = event-data() -> ()  [unwired: 1 in, 1 out]
            n84 = call "NI_USB6343_DO_Port_Mask_Apply.vi"("error in (no error)"=w300, "VI Server Cluster"=w299) -> ("error out"=w298:errorcluster)  [unwired: 9 in]
          }
          event "DO.Port.Update": Value Change {
            n85 = event-data() -> ()  [unwired: 1 in, 1 out]
            n86 = call "NI_USB6343_DO_Port_Update.vi"("error in (no error)"=w303, "VI Server Cluster"=w302) -> ("error out"=w301:errorcluster)  [unwired: 9 in]
          }
          event "EXIT": Value Change {
            n87 = event-data() -> ()  [unwired: 1 in, 1 out]
            n88 = call "NI_USB6343_Accessor_EXIT_Ref.vi"() -> ("EXIT"=w307:refnum<notifier>)  [unwired: 6 in]
            n89 = Send Notification(notification=TRUE, notifier=w307, error in (no error)=w304) -> (error out=w306:errorcluster)  [unwired: 1 out]
          }
          event "FP.Hide": Value Change {
            n90 = event-data() -> ("NewVal"=w308:bool)  [unwired: 1 in]
            n91 = call "NI_USB6343_Accessor_FP_State_Ref.vi"() -> ("FP.State"=w312:refnum<notifier>)  [unwired: 6 in]
            n92 = call "ExecEng_InstrumentsFrontPanel_Hide_Show.vi"("FP.Hide/Show"=w308, "FP.State"=w312, "error in (no error)"=w314, "VI Server Cluster"=w313) -> ("error out"=w310:errorcluster, "VI Server Cluster DUP"=w311:T2)  [unwired: 6 in]
            n93 = call "NI_USB6343_FP_Hide_SendMessageToExecEng.vi"("FP.Open"=w308, "error in (no error)"=w310, "VI Server Cluster"=w311) -> ("error out"=w309:errorcluster)  [unwired: 8 in]
          }
          event "Help": Value Change {
            n94 = event-data() -> ("NewVal"=w315:bool)  [unwired: 1 in]
            n95 = Control Help Window(1:w315) -> ()  [unwired: 1 in]
          }
          event "UDP.ExecEng.Message.String": Shortcut Menu Selection (User) {
            n96 = event-data() -> ("ItemTag"=w319:string)  [unwired: 1 in]
            n97 = case shown="\"Clear Indicator\"" w319 {
              tunnel: w320 -> [w321 w327]
              tunnel: [w321 w326] -> w318
              tunnel: w317 -> [_ w325]
              frame "", Default {
              }
              frame "Clear Indicator" {
                n98 = call-poly "VI Server_Set Control Value.vi"("New Value"="", "Label"="UDP.ExecEng.Message.String" ("Control.Label"), "error in"=w327, "Single Instance (T)"=TRUE ("SingleInstance"), "VI Server Cluster"=w325) -> ("error out"=w326:errorcluster)  [unwired: 4 in, 2 out]
              }
            }
          }
          event "UDP.Responce.String.Monitor": Value Change {
            n99 = event-data() -> ("NewVal"=w328:bool)  [unwired: 1 in]
            n100 = call "NI_USB6343_Accessor_UDP_Responce_String_Monitor_Ref.vi"() -> ("UDP.ExecEng.Command.String.Monitor"=w330:refnum<notifier>)  [unwired: 6 in]
            n101 = Send Notification(notification=w328, notifier=w330, error in (no error)=w331) -> (error out=w329:errorcluster)  [unwired: 1 out]
          }
          event "UDP.Test.String1.Send.ToInstr": Value Change {
            n102 = event-data() -> ()  [unwired: 1 in, 1 out]
            n103 = call-poly "VI Server_GetControl_Value_Ref.vi"("DataType"="", "Control.Label"="UDP.Test.String1", "error in"=w340, "SingleInstance"=TRUE, "VI Server.RefsCluster"=w337) -> ("error out"=w339:errorcluster, "Value"=w332:string)  [unwired: 3 in, 2 out]
            n104 = call "NI_USB6343_Accessor_UDP_Instrument_Responce_Ref.vi"() -> ("UDP.Instrument.Responce.Q"=w333:refnum<queue>)  [unwired: 6 in]
            n105 = Enqueue Element(queue=w333, element=w332, error in (no error)=w339) -> (error out=w338:errorcluster)  [unwired: 1 in, 2 out]
          }
          event "UDP.Test.String1.SendLocal": Value Change {
            n106 = event-data() -> ()  [unwired: 1 in, 1 out]
            n107 = call-poly "VI Server_GetControl_Value_Ref.vi"("DataType"="", "Control.Label"="UDP.Test.String1", "error in"=w349, "SingleInstance"=TRUE, "VI Server.RefsCluster"=w346) -> ("error out"=w348:errorcluster, "Value"=w342:string)  [unwired: 3 in, 2 out]
            n108 = call "NI_USB6343_Accessor_UDP_ExecEng_Instruction_Q_Ref.vi"() -> ("UDP.ExecEng.Instruction.Q"=w341:refnum<queue>)  [unwired: 6 in]
            n109 = Enqueue Element(queue=w341, element=w342, error in (no error)=w348) -> (error out=w347:errorcluster)  [unwired: 1 in, 2 out]
          }
          event "UDP.Test.String2.Send": Value Change {
            n110 = event-data() -> ()  [unwired: 1 in, 1 out]
            n111 = call-poly "VI Server_GetControl_Value_Ref.vi"("DataType"="", "Control.Label"="UDP.Test.String2", "error in"=w358, "SingleInstance"=TRUE, "VI Server.RefsCluster"=w355) -> ("error out"=w357:errorcluster, "Value"=w350:string)  [unwired: 3 in, 2 out]
            n112 = call "NI_USB6343_Accessor_UDP_Instrument_Responce_Ref.vi"() -> ("UDP.Instrument.Responce.Q"=w351:refnum<queue>)  [unwired: 6 in]
            n113 = Enqueue Element(queue=w351, element=w350, error in (no error)=w357) -> (error out=w356:errorcluster)  [unwired: 1 in, 2 out]
          }
          event Timeout {
            n114 = event-data() -> ()  [unwired: 1 in, 1 out]
            n115 = call "NI_USB6343_UserLastSelection_Set_Get_v2.vi"("LoopCounter"=w361, "SynchRefs.Set/Get"=SynchRefs_SetGet."Set", "error in"=w362, "VI Server.RefsCluster"=w360) -> ("error out"=w359:errorcluster)  [unwired: 6 in, 1 out]
          }
        }
        n116 = event shown="[14] \"TestCaseConfiguration\": Shortcut Menu Selection (User)" {
          selector: _ -> [_ _ _ _ _ _ _ _ _ _ _ _ _ _ _ _ _ _ _ _ _ _ _ _]
          dyn-events: _ -> [_ _ _ _ _ _ _ _ _ _ _ _ _ _ _ _ _ _ _ _ _ _ _ _]
          timeout: 250 -> [_ _ _ _ _ _ _ _ _ _ _ _ _ _ _ _ _ _ _ _ _ _ _ _]
          tunnel: w36 -> [w45 w52 w56 w61 w66 w72 w75 w82 w86 w90 w94 w98 w101 w104 _ w107 w110 w113 w116 w119 w123 w128 w132 w135]
          tunnel: [w45 w46 w55 w60 w65 w71 w74 w78 w84 w89 w93 w97 w99 w102 _ w105 w108 w111 w115 w118 w122 w127 w130 w133] -> w33
          tunnel: w32 -> [_ w50 w57 w62 w67 w70 w73 w81 w85 w87 w91 w95 w100 w103 _ w106 w109 w112 _ _ _ _ w131 w134]
          event Timeout {
            n117 = event-data() -> ()  [unwired: 1 in, 1 out]
          }
          event "AI.Physical.Channel", "AI.Sample.Mode", "AI.TerminalConfiguration", "AI.MaxInputLimit", "AI.MinInputLimit", "AI.SampleRate", "AI.Number.Of.Samples", "AI.MultiChannelAcquisition", "AI.Measure", "AI.PhysicalChannel.Include": Value Change {
            n118 = event-data() -> ("CtlRef"=w51:refnum<vi>)  [unwired: 1 in]
            n119 = call "NI_USB6343_Register_User_Last_Action.vi"("CtlRef"=w51, "error in (no error)"=w52, "VI Server Cluster"=w50) -> ("error out"=w47:errorcluster, "VI Server Cluster.DUP"=w48:T2)  [unwired: 7 in]
            n120 = call "NI_USB6343_AI_Configuration_Set_Get.vi"("SynchRefs.Set/Get"=SynchRefs_SetGet."Set", "error in (no error)"=w47, "VI Server Cluster"=w48) -> ("error out"=w46:errorcluster)  [unwired: 6 in, 2 out]
          }
          event "AO.Physical.Channel", "AO.Sample.Clock.Source", "AO.NumberOfSamples", "AO.GenerationMode", "AO.MaxVoltage", "AO.MinVoltage", "AO.SampleRate", "AO.OutputVoltage", "AO.SinewaveFrequency", "AO.Update", "AO.Output": Shortcut Menu Selection (User) {
            n121 = event-data() -> ("CtlRef"=w54:refnum<vi>, "ItemTag"=w53:string)  [unwired: 1 in]
            n122 = call "NI_USB6343_Controls_UserMenu.vi"("ItemTag"=w53, "Control Ref"=w54, "error in (no error)"=w56, "VI Server Cluster"=w57) -> ("error out"=w55:errorcluster)  [unwired: 7 in]
          }
          event "DI.Line", "DI.Line.Update", "DI.Line.State", "DI.Port", "DI.Port.Lines.0:7", "DI.Port.Lines.8:15", "DI.Port.Lines.16:23", "DI.Port.Lines.24:31", "DI.Port.Update", "DO.Line.Update", "DO.Line", "DO.Line.State", "DO.Line.State.Verify", "DO.Port", "DO.Port.Lines.7:0", "DO.Port.Lines.15:8", "DO.Port.Lines.23:16", "DO.Port.Lines.31:24", "DO.Port.Update", "DO.Port.State.Verify", "DO.Port.Lines.7:0.Mask", "DO.Port.Lines.15:8.Mask", "DO.Port.Lines.23:16.Mask", "DO.Port.Lines.31:24.Mask", "DO.Port.Mask.Apply": Shortcut Menu Selection (User) {
            n123 = event-data() -> ("CtlRef"=w59:refnum<vi>, "ItemTag"=w58:string)  [unwired: 1 in]
            n124 = call "NI_USB6343_Controls_UserMenu.vi"("ItemTag"=w58, "Control Ref"=w59, "error in (no error)"=w61, "VI Server Cluster"=w62) -> ("error out"=w60:errorcluster)  [unwired: 7 in]
          }
          event "Cntr.In.Channel", "Cntr.In.Input.Terminal", "Cntr.In.ActiveEdge", "Cntr.In.Sample.Clock.Source", "Cntr.In.IntegrationTime", "Cntr.In.Start", "Cntr.Out.Channel", "Cntr.Out.Output.Terminal", "Cntr.Out.Frequency", "Cntr.Out.Duty.Cycle", "Cntr.Out.Sample.Mode", "Cntr.Out.Start", "Cntr.Out.NumberOfPulses": Shortcut Menu Selection (User) {
            n125 = event-data() -> ("CtlRef"=w64:refnum<vi>, "ItemTag"=w63:string)  [unwired: 1 in]
            n126 = call "NI_USB6343_Controls_UserMenu.vi"("ItemTag"=w63, "Control Ref"=w64, "error in (no error)"=w66, "VI Server Cluster"=w67) -> ("error out"=w65:errorcluster)  [unwired: 7 in]
          }
          event "AI.Physical.Channel", "AI.TerminalConfiguration", "AI.Sample.Mode", "AI.MaxInputLimit", "AI.MinInputLimit", "AI.SampleRate", "AI.Number.Of.Samples", "AI.Measure", "AI.MultiChannelAcquisition", "AI.PhysicalChannel.Include": Shortcut Menu Selection (User) {
            n127 = event-data() -> ("CtlRef"=w69:refnum<vi>, "ItemTag"=w68:string)  [unwired: 1 in]
            n128 = call "NI_USB6343_Controls_UserMenu.vi"("ItemTag"=w68, "Control Ref"=w69, "error in (no error)"=w72, "VI Server Cluster"=w70) -> ("error out"=w71:errorcluster)  [unwired: 7 in]
          }
          event "LastAction.AddToSecuence": Value Change {
            n129 = event-data() -> ()  [unwired: 1 in, 1 out]
            n130 = call "NI_USB6343_UserLastAction_Add_To_Sequence.vi"("error in (no error)"=w75, "VI Server Cluster"=w73) -> ("error out"=w74:errorcluster)  [unwired: 9 in]
          }
          event "AO.Physical.Channel", "AO.MinVoltage", "AO.MaxVoltage", "AO.Sample.Clock.Source", "AO.SampleRate", "AO.NumberOfSamples", "AO.GenerationMode", "AO.SinewaveFrequency", "AO.SampleMode", "AO.OutputVoltage": Value Change {
            n131 = event-data() -> ("CtlRef"=w80:refnum<vi>)  [unwired: 1 in]
            n132 = call "NI_USB6343_Register_User_Last_Action.vi"("CtlRef"=w80, "error in (no error)"=w82, "VI Server Cluster"=w81) -> ("error out"=w79:errorcluster, "VI Server Cluster.DUP"=w77:T2)  [unwired: 7 in]
            n133 = call "NI_USB6343_AO_Configuration_Set_Get.vi"("SynchRefs.Set/Get"=SynchRefs_SetGet."Set", "error in (no error)"=w79, "VI Server Cluster"=w77) -> ("error out"=w78:errorcluster)  [unwired: 6 in, 2 out]
          }
          event "DI.Line", "DI.Port", "DI.Line.Update", "DI.Port.Update": Value Change {
            n134 = event-data() -> ("CtlRef"=w83:refnum<vi>)  [unwired: 1 in]
            n135 = call "NI_USB6343_Register_User_Last_Action_Digital.vi"("CtlRef"=w83, "error in (no error)"=w86, "VI Server Cluster"=w85) -> ("error out"=w84:errorcluster)  [unwired: 8 in]
          }
          event "DO.Line", "DO.Port", "DO.Port.Lines.7:0", "DO.Port.Lines.15:8", "DO.Port.Lines.23:16", "DO.Port.Lines.31:24", "DO.Port.Lines.7:0.Mask", "DO.Port.Lines.15:8.Mask", "DO.Port.Lines.23:16.Mask", "DO.Port.Lines.31:24.Mask", "DO.Port.Update", "DO.Line.Update": Value Change {
            n136 = event-data() -> ("CtlRef"=w88:refnum<vi>)  [unwired: 1 in]
            n137 = call "NI_USB6343_Register_User_Last_Action.vi"("CtlRef"=w88, "error in (no error)"=w90, "VI Server Cluster"=w87) -> ("error out"=w89:errorcluster)  [unwired: 7 in, 1 out]
          }
          event "Cntr.In.Channel", "Cntr.In.Input.Terminal", "Cntr.In.ActiveEdge", "Cntr.In.Sample.Clock.Source", "Cntr.In.IntegrationTime": Value Change {
            n138 = event-data() -> ("CtlRef"=w92:refnum<vi>)  [unwired: 1 in]
            n139 = call "NI_USB6343_Register_User_Last_Action.vi"("CtlRef"=w92, "error in (no error)"=w94, "VI Server Cluster"=w91) -> ("error out"=w93:errorcluster)  [unwired: 7 in, 1 out]
          }
          event "Cntr.Out.Channel", "Cntr.Out.Output.Terminal", "Cntr.Out.Frequency", "Cntr.Out.Duty.Cycle", "Cntr.Out.Sample.Mode", "Cntr.Out.NumberOfPulses": Value Change {
            n140 = event-data() -> ("CtlRef"=w96:refnum<vi>)  [unwired: 1 in]
            n141 = call "NI_USB6343_Register_User_Last_Action.vi"("CtlRef"=w96, "error in (no error)"=w98, "VI Server Cluster"=w95) -> ("error out"=w97:errorcluster)  [unwired: 7 in, 1 out]
          }
          event "TestCase.SAVE": Value Change {
            n142 = event-data() -> ()  [unwired: 1 in, 1 out]
            n143 = call "NI_USB6343_Sequence_Save.vi"("error in (no error)"=w101, "VI Server Cluster"=w100) -> ("error out"=w99:errorcluster)  [unwired: 9 in]
          }
          event "SequenceFile.Open": Value Change {
            n144 = event-data() -> ()  [unwired: 1 in, 1 out]
            n145 = call "NI_USB6343_Sequence_Open.vi"("error in (no error)"=w104, "VI Server Cluster"=w103) -> ("error out"=w102:errorcluster)  [unwired: 9 in]
          }
          event "TestCaseConfiguration": Shortcut Menu Selection (User) {
            n146 = event-data() -> ()  [unwired: 1 in, 2 out]
          }
          event "TestCaseConfiguration": Value Change {
            n147 = event-data() -> ()  [unwired: 1 in, 1 out]
            n148 = call "NI_USB6343_TestCase_Configuration_ValueChanged.vi"("error in"=w107, "VI Server.RefsCluster"=w106) -> ("error out"=w105:errorcluster)  [unwired: 8 in, 1 out]
          }
          event "TestCase.Execute.Selected": Value Change {
            n149 = event-data() -> ()  [unwired: 1 in, 1 out]
            n150 = call "NI_USB6343_ExecuteSelectedInstruction.vi"("error in (no error)"=w110, "VI Server Cluster"=w109) -> ("error out"=w108:errorcluster)  [unwired: 9 in]
          }
          event "TestCase.Execute.All": Value Change {
            n151 = event-data() -> ()  [unwired: 1 in, 1 out]
            n152 = call "NI_USB6343_Execute_All_Instruction.vi"("error in (no error)"=w113, "VI Server Cluster"=w112) -> ("error out"=w111:errorcluster)  [unwired: 9 in]
          }
          event "TestCase.Execute.Pause": Value Change {
            n153 = event-data() -> ("NewVal"=w114:bool)  [unwired: 1 in]
            n154 = call "NI_USB6343_Accessor_Sequence_Execution_Pause_Ref.vi"() -> ("SequenceExecution.PAUSE"=w117:refnum<notifier>)  [unwired: 6 in]
            n155 = Send Notification(notification=w114, notifier=w117, error in (no error)=w116) -> (error out=w115:errorcluster)  [unwired: 1 out]
          }
          event "TestCase.Execute.Next": Value Change {
            n156 = event-data() -> ()  [unwired: 1 in, 1 out]
            n157 = call "NI_USB6343_Accessor_Sequence_Execution_NEXT_Ref.vi"() -> ("SequenceExecution.NEXT"=w121:refnum<notifier>)  [unwired: 6 in]
            n158 = Send Notification(notification=TRUE, notifier=w121, error in (no error)=w119) -> (error out=w118:errorcluster)  [unwired: 1 out]
          }
          event "TestCase.Execute.ABORT": Value Change {
            n159 = event-data() -> ()  [unwired: 1 in, 1 out]
            n160 = call "NI_USB6343_Accessor_Sequence_Execution_ABORT_Ref.vi"() -> ("SequenceExecution.ABORT"=w124:refnum<notifier>)  [unwired: 6 in]
            n161 = Send Notification(notification=TRUE, notifier=w124, error in (no error)=w123) -> (error out=w122:errorcluster)  [unwired: 1 out]
          }
          event "TestCase.Execute.Step.Pause": Value Change {
            n162 = event-data() -> ("NewVal"=w126:bool)  [unwired: 1 in]
            n163 = call "NI_USB6343_TestCase_Execution_Pause_Ref.vi"() -> ("SequenceExecution.StepPAUSE"=w129:refnum<notifier>)  [unwired: 6 in]
            n164 = Send Notification(notification=w126, notifier=w129, error in (no error)=w128) -> (error out=w127:errorcluster)  [unwired: 1 out]
          }
          event "Settings.SAVE": Value Change {
            n165 = event-data() -> ()  [unwired: 1 in, 1 out]
            n166 = call "NI_USB6343_Settings_SAVE.vi"("error in"=w132, "VI Server.RefsCluster"=w131) -> ("error out"=w130:errorcluster)  [unwired: 8 in, 1 out]
          }
          event "Settings.LOAD": Value Change {
            n167 = event-data() -> ()  [unwired: 1 in, 1 out]
            n168 = call "NI_USB6343_Settings_Load.vi"("error in"=w135, "VI Server.RefsCluster"=w134) -> ("error out"=w137:errorcluster, "VI Server.RefsCluster.DUP"=w136:T2)  [unwired: 8 in]
            n169 = call-poly "VI Server_SetControl.vi"("Data"=FALSE, "Control.Label"="Settings.LOAD", "error in"=w137, "SingleInstance"=TRUE, "VI Server.RefsCluster"=w136) -> ("error out"=w133:errorcluster)  [unwired: 4 in, 2 out]
          }
        }
        n170 = call "NI_USB6343_Accessor_EXIT_Ref.vi"() -> ("EXIT"=w38:refnum<notifier>)  [unwired: 6 in]
        n171 = call "Merge Errors II.vi"("error in 2 (no error)"=w33, "error in 1 (no error)"=w35) -> ("error out.DUP"=w34:errorcluster)  [unwired: 4 in, 1 out]
        n172 = call "StopOnErrorOrCommand.vi"("STOP"=w38, "error in (no error)"=w34) -> ("error out"=w40:errorcluster, "STOP"=w39:bool)  [unwired: 8 in]
      }
      n173 = call "NI_USB6343_DAQmx_AI_Measure.vi"("error in (no error)"=w22, "VI Server Cluster"=w20) -> ("error out"=w26:errorcluster)  [unwired: 9 in]
      n174 = call "NI_USB6343_AO_Main_v2.vi"("error in (no error)"=w22, "VI Server Cluster"=w20) -> ("error out"=w23:errorcluster)  [unwired: 9 in]
      n175 = call "NI_USB6343_DAQmx_Counter_IN.vi"("error in (no error)"=w22, "VI Server Cluster"=w20) -> ("error out"=w25:errorcluster)  [unwired: 9 in]
      n176 = call "NI_USB6343_DAQmx_Counter_OUT.vi"("error in (no error)"=w22, "VI Server Cluster"=w20) -> ("error out"=w24:errorcluster)  [unwired: 9 in]
      n177 = call "NI_USB6343_Execute_Instructions_Processor.vi"("error in (no error)"=w22, "VI Server.RefsCluster"=w20) -> ("error out"=w21:errorcluster)  [unwired: 9 in]
      n178 = Build Array(w21, w24, w25, w23, w26, w30) -> (w27:errorcluster[])
      n179 = call "Merge Errors II.vi"("error array in"=w27, "error in 1 (no error)"=w29) -> ("error out.DUP"=w28:errorcluster)  [unwired: 4 in, 1 out]
    }
    frame Error {
    }
  }
  n180 = call-poly "VI Server_GetControl_Value_Ref.vi"("DataType"=tag "" ("DAQmx.Device"), "Control.Label"="DAQmx.Device", "error in"=w13, "SingleInstance"=TRUE, "VI Server.RefsCluster"=w11) -> ("error out"=w16:errorcluster, "Value"=w17:tag, "VI Server.RefsCluster.DUP"=w12:T2)  [unwired: 3 in, 1 out]
  n181 = call <vilib>:"DAQmx Reset Device.vi"("device in"=w17, "error in"=w16) -> ("error out"=w6:errorcluster)  [unwired: 13 in]
  n182 = call "Error _88709_DAQmx_Task Aborted or Device Not Present.vi"("Display Error Message"=FALSE, "error in"=w6) -> ("error out"=w5:errorcluster)  [unwired: 12 in, 1 out]
  n183 = call "VI Server_CloseRefs.vi"("error in"=w5, "VI Server.RefsCluster"=w12) -> ("error out"=w18:errorcluster)  [unwired: 9 in]
  n184 = call "NI_USB6343_Synch_CLOSE.vi"("error in"=w18) -> ("error out"=w9:errorcluster)  [unwired: 10 in]
  n185 = Current VI's Path() -> (path=w7:path)
  n186 = call "Close Window If in EXE mode.vi"("TopLevelVI Path"=w7, "error in"=w9) -> ("error out"=→"error out":errorcluster)  [unwired: 9 in]
